vi "Fetch Waveform.vi"(8 "error in (no error)":errorcluster, 11 "Oscilloscope in":refnum<class "Oscilloscope.lvclass">) -> (0 "error out":errorcluster, 2 "Waveform Data":waveform(dbl)[](graph), 3 "Oscilloscope out":refnum<class "Oscilloscope.lvclass">)   [LabVIEW 2020, in "Oscilloscope.lvclass"]
uses:
  Oscilloscope.lvclass
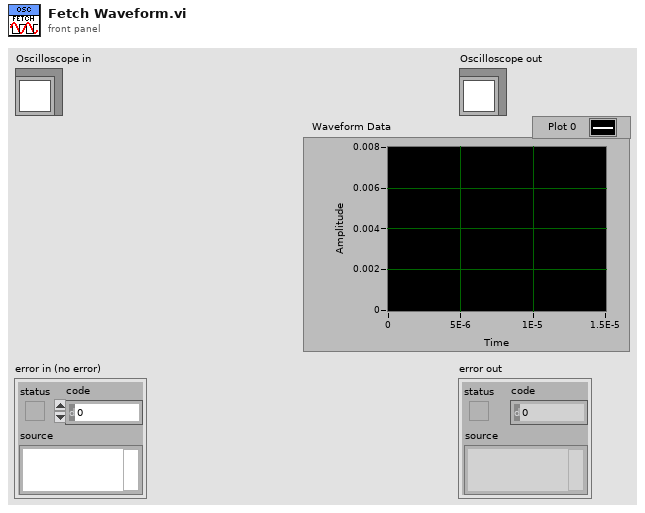
[diagram p1: front panel]
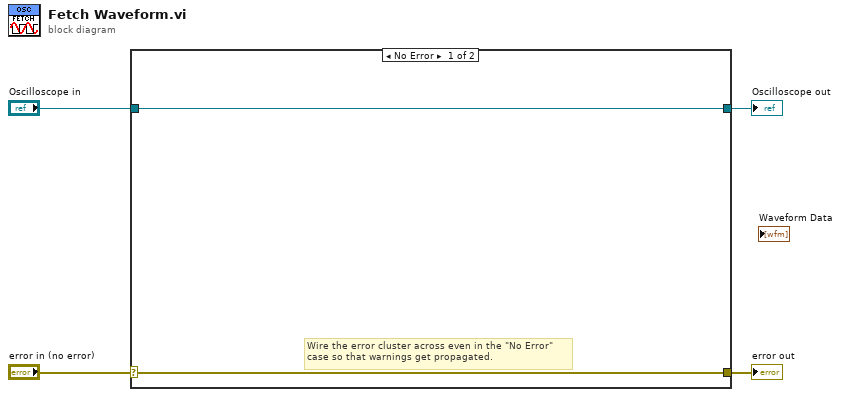
[diagram p0: block diagram]
diagram:
  n1 = case shown="No Error" "error in (no error)" {
    selector: "error in (no error)" -> [w5 w8]
    tunnel: [w5 w8] -> w3
    tunnel: [w6 w7] -> w1
    tunnel: "Oscilloscope in" -> [w6 w7]
    frame No Error {
      # "Wire the error cluster across even in the \"No Error\"\ncase so that warnings get propagated."
    }
    frame Error {
    }
  }
  "error out" <- w3
  "Oscilloscope out" <- w1
